vi "niScope Cal Adjust Compensation Attenuator.vi"(0 "instrument handle":refnum<k15>, 5 "channels":string, 7 "range (V)":dbl format="%.2f", 11 "error in":errorcluster) -> (4 "instrument handle out":refnum<k15>, 15 "error out":errorcluster)   [LabVIEW 2013]
doc: "This VI externally calibrates the compensation attenuator."
uses:
  niScope_32.dll
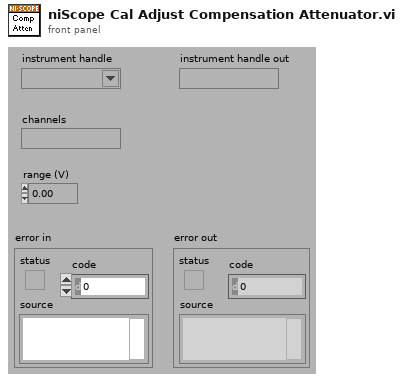
[diagram p1: front panel]
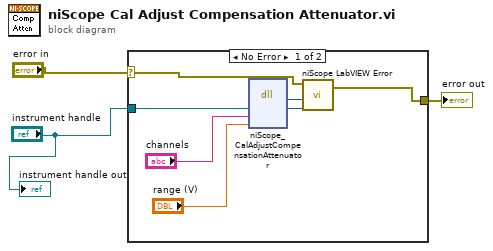
[diagram p0: block diagram]
diagram:
  n1 = case shown="No Error" "error in" {
    selector: "error in" -> [w4 w11]
    tunnel: [w5 w11] -> w3
    tunnel: "instrument handle" -> [w10 _]
    frame No Error {
      n2 = dll-call lib="niScope_*.*" fn="niScope_CalAdjustCompensationAttenuator"("instrumentHandle"=w10, "channelName"="channels", "range"="range (V)") -> (w6:i32, "instrumentHandle"=w7:i32)  [unwired: 5 in, 2 out]
      n3 = call <instrlib>:"niScope LabVIEW Error.vi"("instrument handle"=w7, "niScope error code (0)"=w6, "error in (no error)"=w4) -> ("error out"=w5:errorcluster)  [unwired: 2 in]
    }
    frame Error {
    }
  }
  "error out" <- w3
  "instrument handle out" <- "instrument handle"
